vi "data_proc.vi"(8 "error out 2":errorcluster, 10 "gui_q":refnum<queue>, 11 "data_q":refnum<queue>) -> (0 "error out":errorcluster)   [LabVIEW 2023]
uses:
  Labview/img_data.ctl
  <vilib>/picture/picture.llb/imagedata.ctl
  Labview/data_commands.ctl
  Labview/data.ctl
  Labview/commands.ctl
  <vilib>/Analysis/2dsp.llb/2D Convolution (DBL).vi
  <vilib>/Analysis/NI_AALPro.lvlib
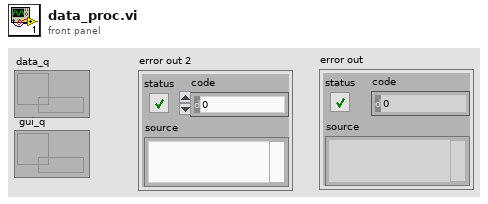
[diagram p1: front panel]
types:
  T1 = typedef "data.ctl" = cluster{"gui_commands":T2, "curent":T3, "ori":T3}
  T2 = typedef "commands.ctl" = enum16{"display", "bin", "gauss", "edg", "blurr", "connect", "stop", "idle"}
  T3 = typedef "imagedata.ctl" = cluster{"image type":i32, "image depth":i32, "image":u8[], "mask":u8[], "colors":u32[], "Rectangle":cluster{"left":i16, "top":i16, "right":i16, "bottom":i16}}
  T4 = typedef "img_data.ctl" = cluster{"ori":T3, "curent":T3, "comands":T5}
  T5 = typedef "data_commands.ctl" = enum16{"stop", "bin", "edg", "gauss", "blurr", "idle"}
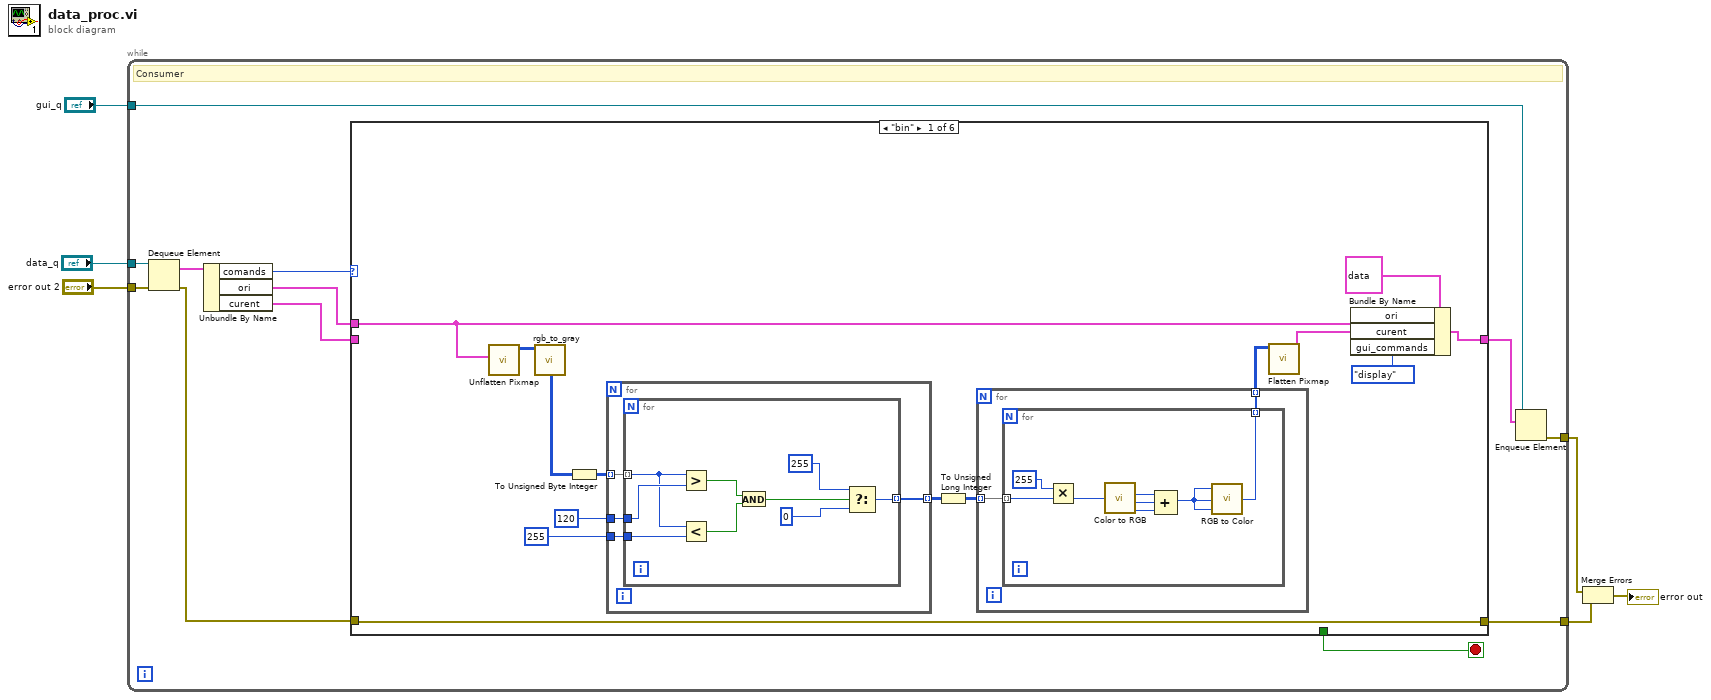
[diagram p0: block diagram]
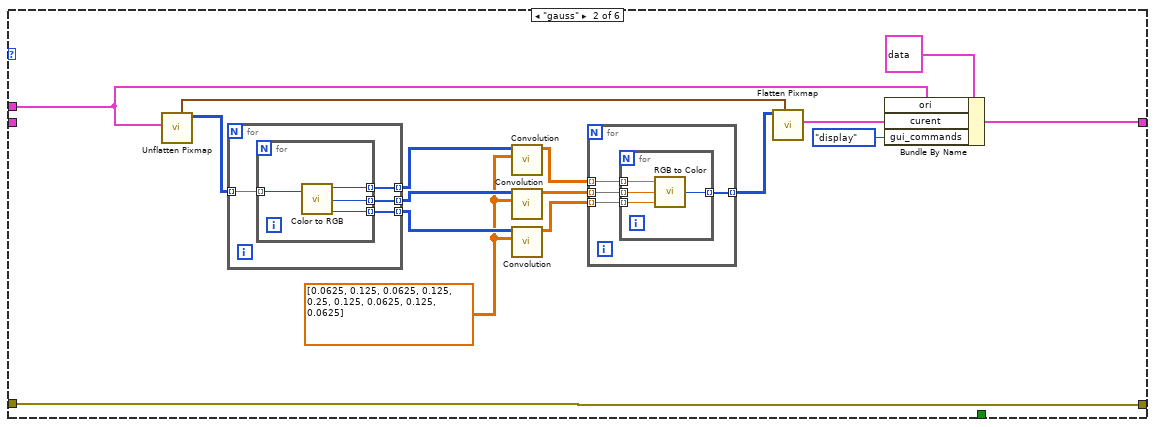
[diagram p2: hidden frame]
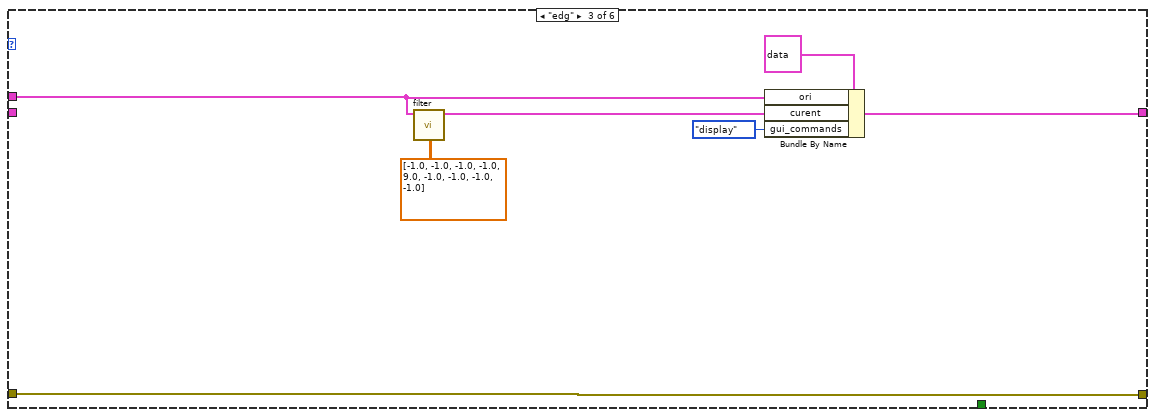
[diagram p3: hidden frame]
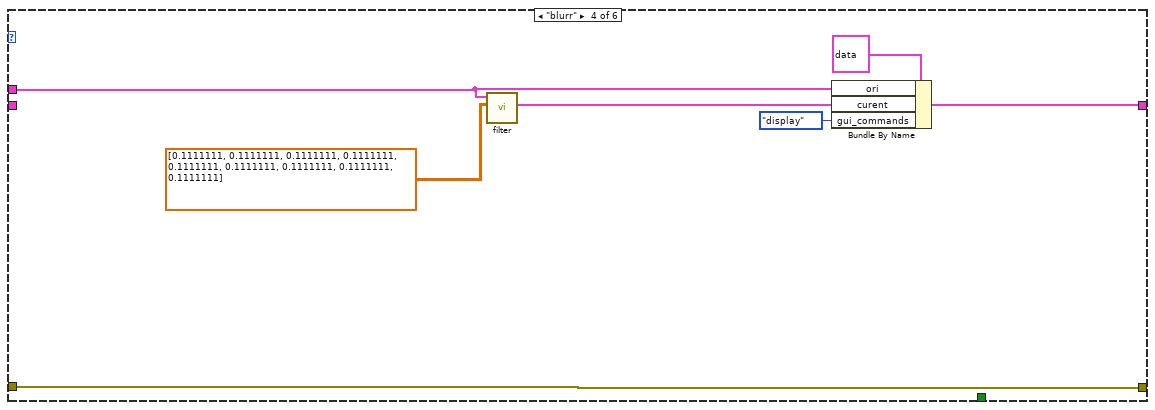
[diagram p4: hidden frame]
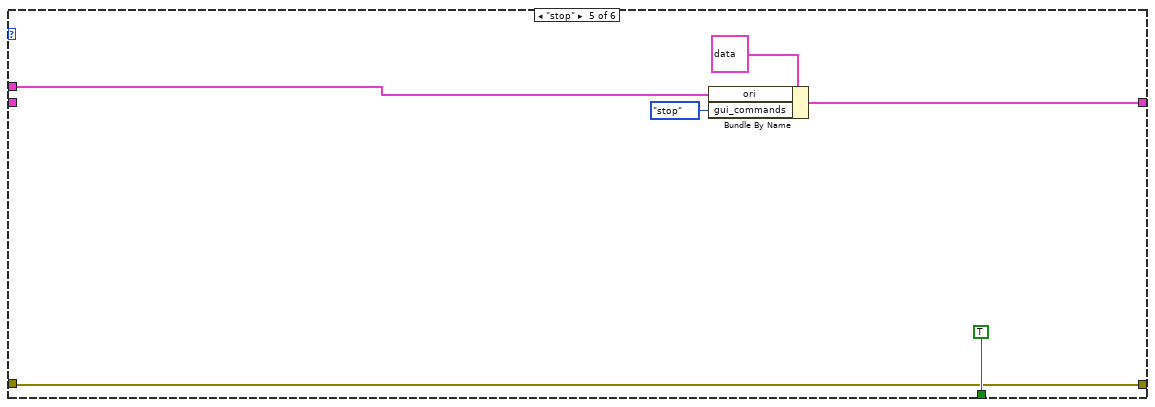
[diagram p5: hidden frame]
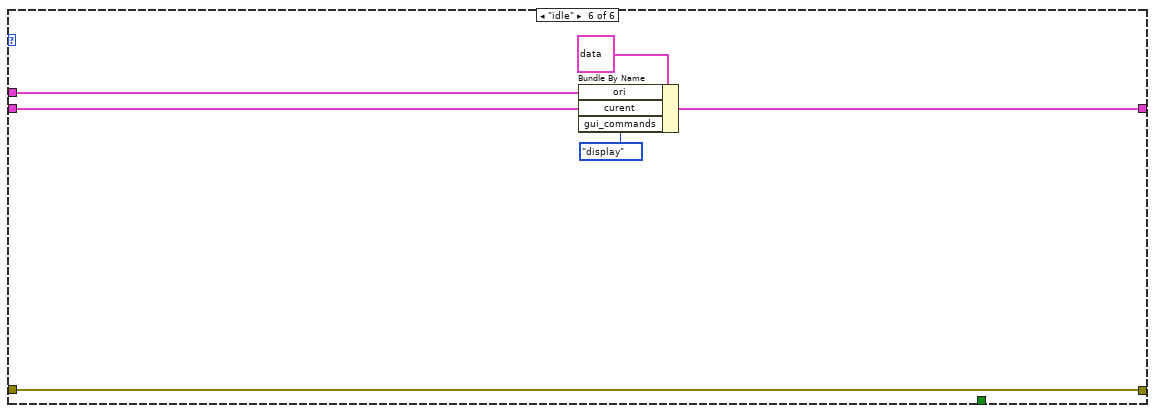
[diagram p6: hidden frame]
diagram:
  n1 = while {
    tunnel: [w17] -> w5
    tunnel: "data_q" -> [w16]
    tunnel: "error out 2" -> [w15]
    tunnel: [w14] -> w3
    tunnel: "gui_q" -> [w9]
    stop <- w18 stop-if-true
    # "Consumer"
    n2 = Dequeue Element(queue=w16, error in (no error)=w15) -> (element=w12:T4, error out=w13:errorcluster)  [unwired: 1 in, 2 out]
    n3 = Unbundle By Name(w12) -> ("comands"=w11:T5, "ori"=w10:T3, "curent"=w7:T3)
    n4 = case shown="\"bin\"" w11 {
      tunnel: [_ _ _ _ TRUE _] -> w18
      tunnel: w13 -> [w30 w60 w92 w101 w106 w113]
      tunnel: [w30 w60 w92 w101 w106 w113] -> w17
      tunnel: w10 -> [w22 w59 w91 w98 w105 w111]
      tunnel: [w20 w58 w88 w97 w104 w110] -> w8
      tunnel: w7 -> [_ _ _ _ _ w109]
      frame "bin" {
        n5 = call <vilib>:"Unflatten Pixmap.vi"("image data"=w22) -> ("24-bit pixmap"=w32:u32[][])  [unwired: 4 in, 6 out]
        n6 = call "rgb_to_gray.vi"("24-bit pixmap"=w32) -> ("Array"=w29:u32[][])  [unwired: 10 in]
        n7 = To Unsigned Byte Integer(number=w29) -> (unsigned 8bit integer=w26:u8[][])
        n8 = for {
          tunnel: w26 -> [w46] mode=indexing
          tunnel: u8 120 ("Threshold min") -> [w45]
          tunnel: u8 255 ("Threshold max") -> [w44]
          tunnel: [w43] -> w24 mode=indexing
          n9 = for {
            tunnel: w46 -> [w53] mode=indexing
            tunnel: w45 -> [w55]
            tunnel: w44 -> [w54]
            tunnel: [w47] -> w43 mode=indexing
            n10 = Greater?(x=w53, y=w55) -> (0:w52:bool)
            n11 = Less?(x=w53, y=w54) -> (x < y?=w51:bool)
            n12 = And(x=w52, y=w51) -> (x .and. y?=w50:bool)
            n13 = Select(t=u32 255, s=w50, f=u32 0) -> (s? t:f=w47:u32)
          }
        }
        n14 = To Unsigned Long Integer(number=w24) -> (unsigned 32bit integer=w25:u32[][])
        n15 = for {
          tunnel: w25 -> [w34] mode=indexing
          tunnel: [w33] -> w23 mode=indexing
          n16 = for {
            tunnel: w34 -> [w42] mode=indexing
            tunnel: [w37] -> w33 mode=indexing
            n17 = Multiply(x=u32 255, y=w42) -> (x*y=w36:u32)
            n18 = call <vilib>:"Color to RGB.vi"("Color"=w36) -> ("R"=w41:u8, "G"=w40:u8, "B"=w39:u8)  [unwired: 1 out]
            n19 = Compound Arithmetic op=ADD(w41, w40, w39) -> (w38:u8)
            n20 = call <vilib>:"RGB to Color.vi"("B"=w38, "G"=w38, "R"=w38) -> ("Color"=w37:u32)
          }
        }
        n21 = call <vilib>:"Flatten Pixmap.vi"("24-bit pixmap"=w23) -> ("image data"=w31:T3)  [unwired: 10 in]
        n22 = Bundle By Name(cluster=T1 {"gui_commands"=enum."bin", "curent"={"image type"=0, "image depth"=0, "image"=[], "mask"=[], "colors"=[], "Rectangle"={"left"=0, "top"=0, "right"=0, "bottom"=0}}, "ori"={"image type"=0, "image depth"=0, "image"=[], "mask"=[], "colors"=[], "Rectangle"={"left"=0, "top"=0, "right"=0, "bottom"=0}}} ("gui_data"), "ori"=w22, "curent"=w31, "gui_commands"=commands."display") -> (w20:T1)
      }
      frame "gauss" {
        w62 = dbl[][] [[0.0625, 0.125, 0.0625], [0.125, 0.25, 0.125], [0.0625, 0.125, 0.0625]] ("Array")
        n23 = call <vilib>:"Unflatten Pixmap.vi"("image data"=w59) -> ("24-bit pixmap"=w64:u32[][], "top left"=w63:cluster{"x":i16, "y":i16})  [unwired: 4 in, 5 out]
        n24 = for {
          tunnel: w64 -> [w83] mode=indexing
          tunnel: [w82] -> w65 mode=indexing
          tunnel: [w81] -> w66 mode=indexing
          tunnel: [w80] -> w67 mode=indexing
          n25 = for {
            tunnel: w83 -> [w87] mode=indexing
            tunnel: [w86] -> w82 mode=indexing
            tunnel: [w85] -> w81 mode=indexing
            tunnel: [w84] -> w80 mode=indexing
            n26 = call <vilib>:"Color to RGB.vi"("Color"=w87) -> ("R"=w86:u8, "G"=w85:u8, "B"=w84:u8)  [unwired: 1 out]
          }
        }
        n27 = call-poly <vilib>:"Convolution.vi"("Y"=w62, "X"=w65) -> ("X * Y"=w68:dbl[][])  [unwired: 8 in, 1 out]
        n28 = call-poly <vilib>:"Convolution.vi"("Y"=w62, "X"=w66) -> ("X * Y"=w69:dbl[][])  [unwired: 8 in, 1 out]
        n29 = call-poly <vilib>:"Convolution.vi"("Y"=w62, "X"=w67) -> ("X * Y"=w70:dbl[][])  [unwired: 8 in, 1 out]
        n30 = for {
          tunnel: w68 -> [w75] mode=indexing
          tunnel: w69 -> [w74] mode=indexing
          tunnel: w70 -> [w73] mode=indexing
          tunnel: [w72] -> w71 mode=indexing
          n31 = for {
            tunnel: w75 -> [w79] mode=indexing
            tunnel: w74 -> [w78] mode=indexing
            tunnel: w73 -> [w77] mode=indexing
            tunnel: [w76] -> w72 mode=indexing
            n32 = call <vilib>:"RGB to Color.vi"("B"=w77, "G"=w78, "R"=w79) -> ("Color"=w76:u32)
          }
        }
        n33 = call <vilib>:"Flatten Pixmap.vi"("top left"=w63, "24-bit pixmap"=w71) -> ("image data"=w61:T3)  [unwired: 9 in]
        n34 = Bundle By Name(cluster=T1 {"gui_commands"=enum."bin", "curent"={"image type"=0, "image depth"=0, "image"=[], "mask"=[], "colors"=[], "Rectangle"={"left"=0, "top"=0, "right"=0, "bottom"=0}}, "ori"={"image type"=0, "image depth"=0, "image"=[], "mask"=[], "colors"=[], "Rectangle"={"left"=0, "top"=0, "right"=0, "bottom"=0}}} ("gui_data"), "ori"=w59, "curent"=w61, "gui_commands"=commands."display") -> (w58:T1)
      }
      frame "edg" {
        n35 = call "filter.vi"("Array"=dbl[][] [[-1.0, -1.0, -1.0], [-1.0, 9.0, -1.0], [-1.0, -1.0, -1.0]], "ori"=w91) -> ("image data"=w94:T3)  [unwired: 9 in]
        n36 = Bundle By Name(cluster=T1 {"gui_commands"=enum."bin", "curent"={"image type"=0, "image depth"=0, "image"=[], "mask"=[], "colors"=[], "Rectangle"={"left"=0, "top"=0, "right"=0, "bottom"=0}}, "ori"={"image type"=0, "image depth"=0, "image"=[], "mask"=[], "colors"=[], "Rectangle"={"left"=0, "top"=0, "right"=0, "bottom"=0}}} ("gui_data"), "ori"=w91, "curent"=w94, "gui_commands"=commands."display") -> (w88:T1)
      }
      frame "blurr" {
        n37 = call "filter.vi"("Array"=dbl[][] [[0.1111111, 0.1111111, 0.1111111], [0.1111111, 0.1111111, 0.1111111], [0.1111111, 0.1111111, 0.1111111]], "ori"=w98) -> ("image data"=w99:T3)  [unwired: 9 in]
        n38 = Bundle By Name(cluster=T1 {"gui_commands"=enum."bin", "curent"={"image type"=0, "image depth"=0, "image"=[], "mask"=[], "colors"=[], "Rectangle"={"left"=0, "top"=0, "right"=0, "bottom"=0}}, "ori"={"image type"=0, "image depth"=0, "image"=[], "mask"=[], "colors"=[], "Rectangle"={"left"=0, "top"=0, "right"=0, "bottom"=0}}} ("gui_data"), "ori"=w98, "curent"=w99, "gui_commands"=commands."display") -> (w97:T1)
      }
      frame "stop" {
        n39 = Bundle By Name(cluster=T1 {"gui_commands"=enum."bin", "curent"={"image type"=0, "image depth"=0, "image"=[], "mask"=[], "colors"=[], "Rectangle"={"left"=0, "top"=0, "right"=0, "bottom"=0}}, "ori"={"image type"=0, "image depth"=0, "image"=[], "mask"=[], "colors"=[], "Rectangle"={"left"=0, "top"=0, "right"=0, "bottom"=0}}} ("gui_data"), "ori"=w105, "gui_commands"=commands."stop") -> (w104:T1)
      }
      frame "idle" {
        n40 = Bundle By Name(cluster=T1 {"gui_commands"=enum."bin", "curent"={"image type"=0, "image depth"=0, "image"=[], "mask"=[], "colors"=[], "Rectangle"={"left"=0, "top"=0, "right"=0, "bottom"=0}}, "ori"={"image type"=0, "image depth"=0, "image"=[], "mask"=[], "colors"=[], "Rectangle"={"left"=0, "top"=0, "right"=0, "bottom"=0}}} ("gui_data"), "ori"=w111, "curent"=w109, "gui_commands"=commands."display") -> (w110:T1)
      }
    }
    n41 = Enqueue Element(queue=w9, element=w8) -> (error out=w14:errorcluster)  [unwired: 2 in, 2 out]
  }
  n42 = Merge Errors(w3, w5) -> (→"error out":errorcluster)
